vi "init_hw.vi"(8 "error in (no error)":errorcluster, 11 "ESP301viaTCPIP in":refnum<class "ESP301viaTCPIP.lvclass">) -> (0 "error out":errorcluster, 2 "Boolean":bool=TRUE, 3 "ESP301viaTCPIP out":refnum<class "ESP301viaTCPIP.lvclass">)   [LabVIEW 2019, in "ESP301viaTCPIP.lvlib" / "ESP301viaTCPIP.lvclass"]
uses:
  ESP301viaTCPIP.lvclass
  ESP301viaTCPIP.lvlib
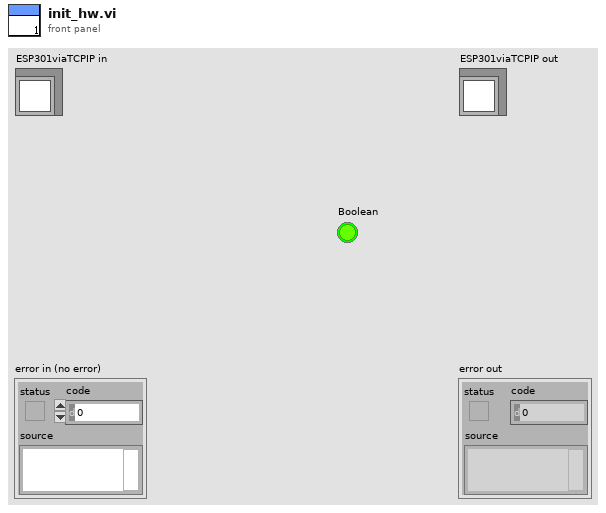
[diagram p1: front panel]
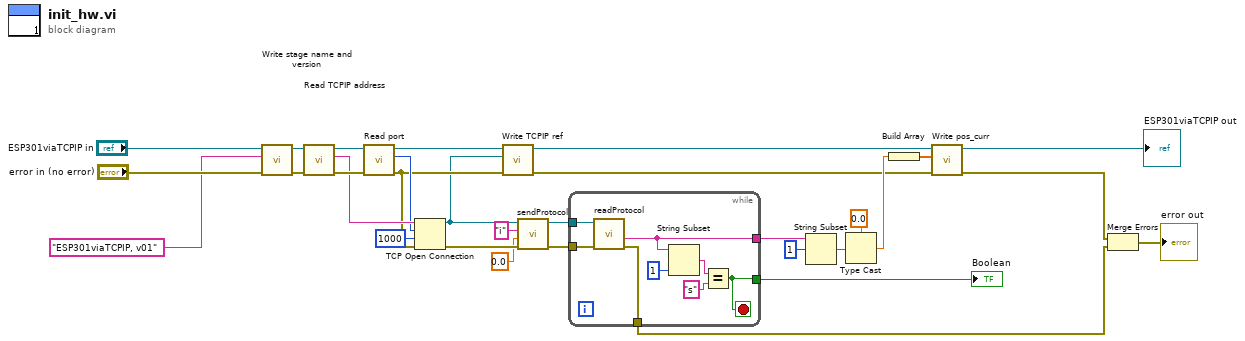
[diagram p0: block diagram]
diagram:
  n1 = call-dynamic "Write stage name and version.vi"("error in (no error)"="error in (no error)", "stage name and version"="ESP301viaTCPIP, v01", "_stage in"="ESP301viaTCPIP in") -> ("error out"=w27:errorcluster, "_stage out"=w28:refnum<class "ESP301viaTCPIP.lvclass">)  [unwired: 7 in]
  n2 = call-dynamic "Read TCPIP address.vi"("error in (no error)"=w27, "ESP301viaTCPIP in"=w28) -> ("error out"=w25:errorcluster, "TCPIP address"=w24:string, "ESP301viaTCPIP out"=w26:refnum<class "ESP301viaTCPIP.lvclass">)  [unwired: 7 in]
  n3 = call-dynamic "Read port.vi"("error in (no error)"=w25, "ESP301viaTCPIP in"=w26) -> ("error out"=w20:errorcluster, "port"=w23:u16, "ESP301viaTCPIP out"=w21:refnum<class "ESP301viaTCPIP.lvclass">)  [unwired: 7 in]
  n4 = TCP Open Connection(address=w24, remote port or service name=w23, timeout ms (60000)=1000, error in (no error)=w20) -> (connection ID=w18:refnum<k5>, error out=w17:errorcluster)  [unwired: 1 in]
  n5 = call-dynamic "Write TCPIP ref.vi"("error in (no error)"=w20, "TCPIP ref"=w18, "ESP301viaTCPIP in"=w21) -> ("error out"=w2:errorcluster, "ESP301viaTCPIP out"=w5:refnum<class "ESP301viaTCPIP.lvclass">)  [unwired: 7 in]
  n6 = call "sendProtocol.vi"("error in (no error)"=w17, "GoTo position"=0.0, "command"="i", "TCP Network Connection in"=w18) -> ("error out"=w13:errorcluster, "TCP Network Connection out"=w14:refnum<k5>)  [unwired: 6 in]
  n7 = while {
    tunnel: w14 -> [w39]
    tunnel: w13 -> [w38]
    tunnel: [w35] -> w7
    tunnel: [w34] -> w9
    tunnel: [w33] -> w6
    stop <- w35 stop-if-true
    n8 = call "readProtocol.vi"("error in (no error)"=w38, "TCP Network Connection in"=w39) -> ("error out"=w33:errorcluster, "data out"=w34:string)  [unwired: 8 in]
    n9 = String Subset(string=w34, length (rest)=1 ("offset (0)")) -> (substring=w37:string)  [unwired: 1 in]
    n10 = Equal?(x=w37, y="s") -> (x = y?=w35:bool)
  }
  "Boolean" <- w7
  n11 = String Subset(string=w9, offset (0)=1) -> (substring=w12:string)  [unwired: 1 in]
  n12 = Type Cast(type=0.0, x=w12) -> (*(type *) &x=w8:dbl)
  n13 = Build Array(w8) -> (w1:dbl[])
  n14 = call-dynamic "Write pos_curr.vi"("error in (no error)"=w2, "set_pos"=w1, "_stage in"=w5) -> ("error out"=w3:errorcluster, "_stage out"=→"ESP301viaTCPIP out":refnum<class "ESP301viaTCPIP.lvclass">)  [unwired: 7 in]
  n15 = Merge Errors(w3, w6) -> (→"error out":errorcluster)
